vi "IBM4_Write.vi"(8 "error in":errorcluster, 9 "Vset":dbl=1.0, 10 "Channel":i32, 11 "COM resource in":refnum<visa-resource-name>="COM9") -> (0 "error out":errorcluster, 3 "COM resource out":refnum<visa-resource-name>)   [LabVIEW 2022 SP3, in "IBM4.lvlib"]
doc: "This VI interfaces with the IBM4 to perform a write operation where a Voltage is output on one of the analogue output pins of the IBM4.\n\nThe output channel must be 0 or 1, while the output value should be specified in Volts (thus, floating point)"
uses:
  <instrlib>/IBM4/IBM4.lvlib
panel:
  out "read buffer":string
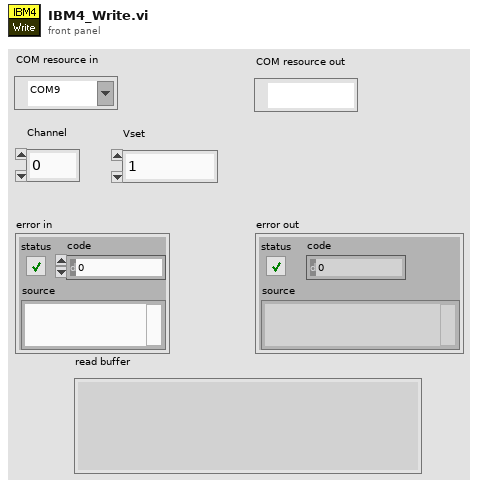
[diagram p1: front panel]
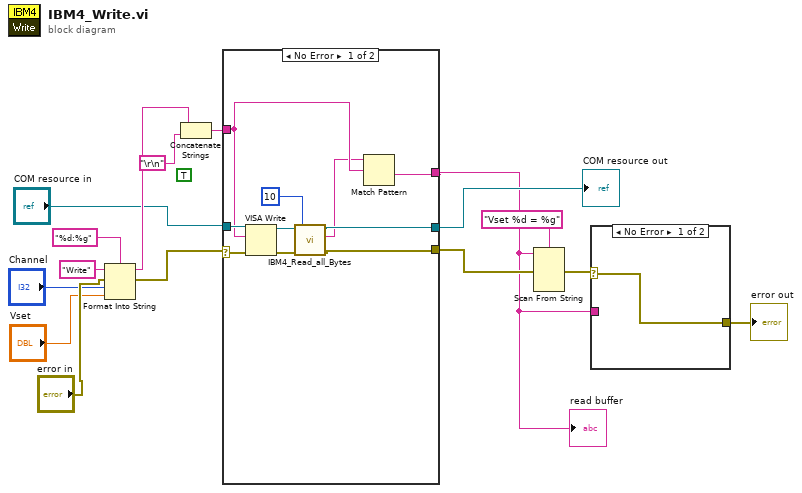
[diagram p0: block diagram]
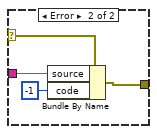
[diagram p2: hidden frame]
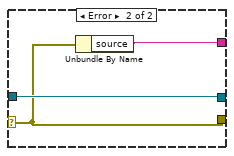
[diagram p3: hidden frame]
diagram:
  (unwired) TRUE ("Enable Termination\nChar (T)")
  n1 = Format Into String(format string="%d:%g", initial string="Write", error in="error in", "Channel", "Vset") -> (resulting string=w7:string, error out=w1:errorcluster)
  n2 = Concatenate Strings(w7, "\r\n") -> (w6:string)
  n3 = case shown="No Error" w1 {
    selector: w1 -> [w23 w27]
    tunnel: "COM resource in" -> [w26 w29]
    tunnel: [w18 w27] -> w10
    tunnel: [w25 w28] -> w3
    tunnel: w6 -> [w24 _]
    tunnel: [w19 w29] -> w11
    frame No Error {
      n4 = VISA Write(VISA resource name=w26, write buffer=w24, error in (no error)=w23) -> (VISA resource name out=w22:refnum<visa-resource-name>, error out=w21:errorcluster)  [unwired: 1 out]
      n5 = call <instrlib>:"IBM4_Read_all_Bytes.vi"("error in (no error)"=w21, "milliseconds to wait"=u32 10, "VISA Refnum in"=w22) -> ("error out"=w18:errorcluster, "String"=w17:string, "VISA Refnum out"=w19:refnum<visa-resource-name>)  [unwired: 2 in]
      n6 = Match Pattern(string=w17, regular expression=w24) -> (after substring=w25:string)  [unwired: 1 in, 3 out]
    }
    frame Error {
      n7 = Unbundle By Name(w27) -> ("source"=w28:string)
    }
  }
  "COM resource out" <- w11
  "read buffer" <- w3
  n8 = Scan From String(format string="Vset %d = %g", input string=w3, error in=w10) -> (error out=w5:errorcluster)  [unwired: 5 in, 2 out]
  n9 = case shown="No Error" w5 {
    selector: w5 -> [w30 w34]
    tunnel: [w30 w32] -> w4
    tunnel: w3 -> [_ w33]
    frame No Error {
    }
    frame Error {
      n10 = Bundle By Name(cluster=w34, "source"=w33, "code"=-1) -> (w32:errorcluster)
    }
  }
  "error out" <- w4
